vi "Generate Unique File Name.vi"(8 "error in":errorcluster, 11 "File Actor in":refnum<class "File Actor.lvclass">) -> (0 "error out":errorcluster, 2 "File Name":string, 3 "File Actor out":refnum<class "File Actor.lvclass">)   [LabVIEW 2014, in "File Library.lvlib" / "File Actor.lvclass"]
uses:
  File Actor.lvclass
  File Actor.lvclass/File Actor.ctl
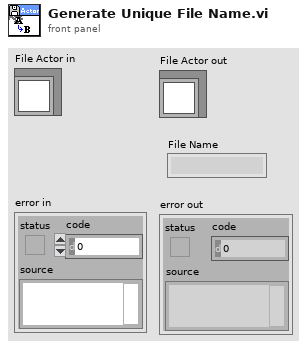
[diagram p1: front panel]
types:
  T1 = typedef "LVDateTimeRec.ctl" = cluster{"fractional second":dbl, "second":i32, "minute":i32, "hour":i32, "day of month":i32, "month":i32, "year":i32, "day of week":i32, "day of year":i32, "DST":i32}
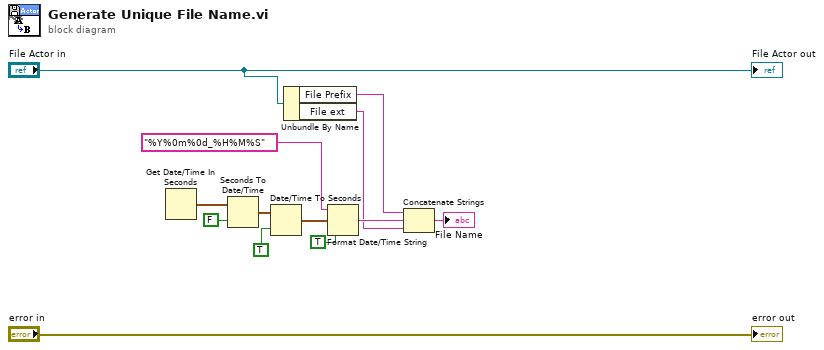
[diagram p0: block diagram]
diagram:
  n1 = Get Date/Time In Seconds() -> (seconds since 1Jan1904=w9:timestamp)
  n2 = Seconds To Date/Time(time stamp (now)=w9, to UTC (F)=FALSE) -> (date time rec=w6:T1)
  n3 = Date/Time To Seconds(1:TRUE ("is UTC (F)"), 2:w6) -> (0:w5:timestamp)
  n4 = Unbundle By Name("File Actor in") -> ("File Prefix"=w3:string, "File ext"=w4:string)
  n5 = Format Date/Time String(time format string (%c)="%Y%0m%0d_%H%M%S", seconds (now)=w5, UTC format=TRUE) -> (date/time string=w10:string)
  n6 = Concatenate Strings(w3, w10, w4) -> (→"File Name":string)
  "error out" <- "error in"
  "File Actor out" <- "File Actor in"
